vi "Logic for Default Case - Single Converter.vi"(11 "error in":errorcluster) -> (15 "error out":errorcluster)   [LabVIEW 2021, in "Converter.lvlib"]
uses:
  <vilib>/Utility/traverseref.llb/TRef TravTarget.ctl
  Converter.lvlib
  <vilib>/Utility/traverseref.llb/VI Scripting - Traverse.lvlib
  Converter Reusables/Converter Reusables.lvlib
  Path Functions/Path Functions.lvlib
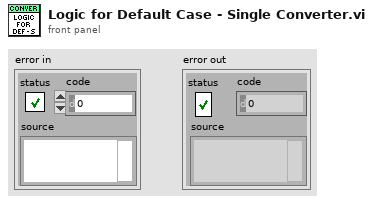
[diagram p1: front panel]
types:
  T1 = typedef "TRef TravTarget.ctl" = enum16{"FP", "BD", "Other"}
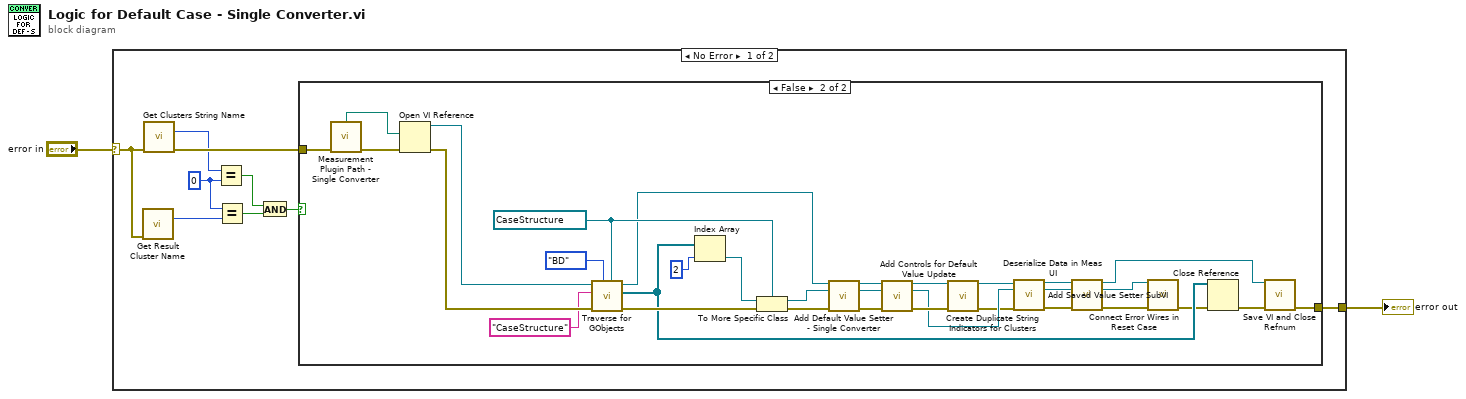
[diagram p0: block diagram]
diagram:
  n1 = case shown="No Error" "error in" {
    selector: "error in" -> [w10 w45]
    tunnel: [w11 w45] -> w2
    frame No Error {
      w4 = 0 ("y")
      n2 = call "Get Result Cluster Name.vi"("error in"=w10) -> ("array size"=w7:i32)  [unwired: 12 in, 2 out]
      n3 = call "Get Clusters String Name.vi"("error in"=w10) -> ("array size"=w8:i32, "error out"=w9:errorcluster)  [unwired: 12 in, 1 out]
      n4 = Equal?(x=w8, y=w4) -> (x = y?=w6:bool)
      n5 = Equal?(x=w4, y=w7) -> (x = y?=w3:bool)
      n6 = And(x=w6, y=w3) -> (x .and. y?=w5:bool)
      n7 = case shown="False" w5 {
        tunnel: [w12 w39] -> w11
        tunnel: w9 -> [w12 w21]
        frame True {
        }
        frame False {
          w41 = refnum<vi> refnum ("Other Refnum")
          n8 = call "Measurement Plugin Path - Single Converter.vi"("error in"=w21) -> ("measurement ui"=w23:path, "error out"=w22:errorcluster)  [unwired: 2 in, 11 out]
          n9 = Open VI Reference(vi path=w23, error in (no error)=w22) -> (vi reference=w35:refnum<vi>, error out=w44:errorcluster)  [unwired: 4 in]
          n10 = call <vilib>:"Traverse for GObjects.vi"("Other Refnum"=w41, "Traverse Target"=TRef_TravTarget."BD", "error in (no error)"=w44, "Class Name"="CaseStructure", "VI Refnum"=w35) -> ("error out"=w40:errorcluster, "References"=w29:refnum<vi>[], "dup VI Refnum"=w20:refnum<vi>)  [unwired: 3 in, 1 out]
          n11 = Index Array(array=w29, index=2) -> (element=w37:refnum<vi>)
          n12 = To More Specific Class(target class=w41, reference=w37, error in=w40) -> (specific class reference=w19:refnum<vi>, error out=w18:errorcluster)
          n13 = call "Add Default Value Setter - Single Converter.vi"("vi in"=w20, "case sel refnum"=w19, "error in"=w18) -> ("vi out"=w16:refnum<vi>, "case sel refnum out"=w15:refnum<vi>, "error out"=w17:errorcluster)  [unwired: 10 in]
          n14 = call "Add Controls for Default Value Update.vi"("vi refnum"=w16, "case sel refnum"=w15, "error in"=w17) -> ("vi refnum out"=w34:refnum<vi>, "case sel refnum out"=w32:refnum<vi>, "error out"=w36:errorcluster)  [unwired: 10 in]
          n15 = call "Create Duplicate String Indicators for Clusters.vi"("ui vi ref"=w34, "error in"=w36) -> ("ui vi ref out"=w33:refnum<vi>, "error out"=w26:errorcluster)  [unwired: 12 in]
          n16 = call "Add Saved Value Setter SubVI.vi"("vi in"=w33, "case sel refnum in"=w32, "error in"=w26) -> ("vi out"=w31:refnum<vi>, "case sel refnum out"=w30:refnum<vi>, "error out"=w27:errorcluster)  [unwired: 10 in]
          n17 = call "Deserialize Data in Meas UI.vi"("vi refnum in"=w31, "case sel refnum in"=w30, "error in"=w27) -> ("vi refnum out"=w13:refnum<vi>, "case sel refnum out"=w14:refnum<vi>, "error out"=w24:errorcluster)  [unwired: 10 in]
          n18 = call "Connect Error Wires in Reset Case.vi"("case sel refnum in"=w14, "error in"=w24) -> ("error out"=w25:errorcluster)  [unwired: 12 in, 1 out]
          n19 = Close Reference(reference=w29, error in (no error)=w25) -> (error out=w28:errorcluster)
          n20 = call "Save VI and Close Refnum.vi"("vi refnum"=w13, "error in"=w28) -> ("error out"=w39:errorcluster)  [unwired: 13 in]
        }
      }
    }
    frame Error {
    }
  }
  "error out" <- w2
